vi "SetupControls.vi"(8 "Error IN":errorcluster, 11 "hCamera IN":u32) -> (0 "Error OUT":errorcluster, 3 "hCamera OUT":u32)   [LabVIEW 2013]
uses:
  Controls/Control References.ctl
  <vilib>/addons/PixeLINK/Low Level Functions/CAMERA_FEATURES.llb/TDPU-CameraFeatures-PixelAddressingMode.ctl
panel:
  in  "Camera Control References":T1
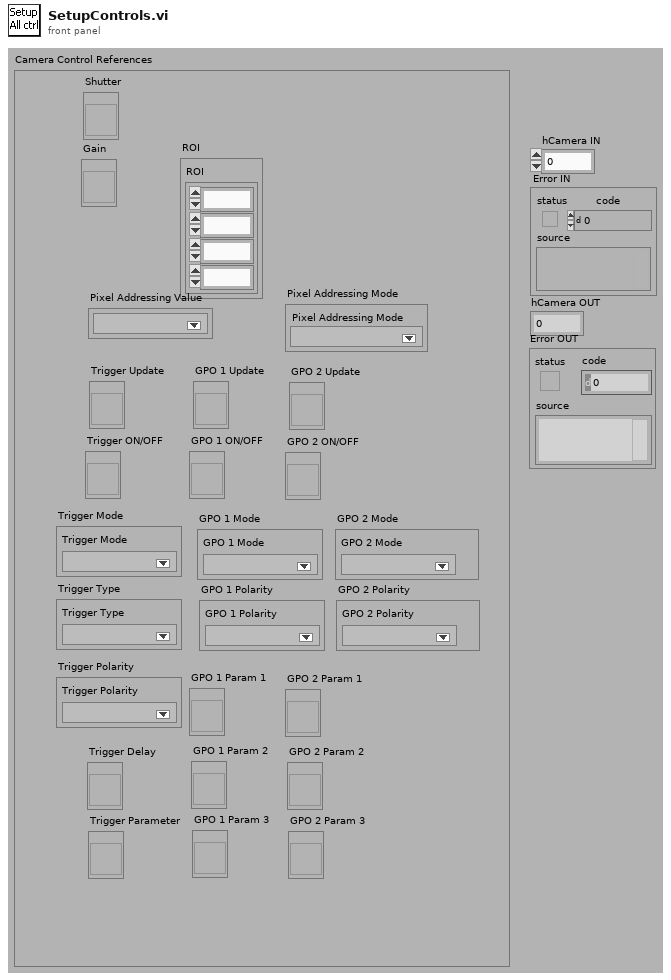
[diagram p1: front panel]
types:
  T1 = typedef "Control References.ctl" = cluster{"Shutter":refnum<vi>, "Gain":refnum<vi>, "ROI":refnum<vi>, "Pixel Addressing Value":refnum<vi>, "Trigger ON/OFF":refnum<vi>, "Trigger Mode":refnum<vi>, "Trigger Type":refnum<vi>, "Trigger Polarity":refnum<vi>, "Trigger Delay":refnum<vi>, "Trigger Parameter":refnum<vi>, "GPO 1 Mode":refnum<vi>, "GPO 1 Polarity":refnum<vi>, "GPO 1 Param 2":refnum<vi>, "GPO 1 Param 3":refnum<vi>, "GPO 1 Param 1":refnum<vi>, "GPO 1 ON/OFF":refnum<vi>, "GPO 2 Mode":refnum<vi>, "GPO 2 Polarity":refnum<vi>, "GPO 2 Param 2":refnum<vi>, "GPO 2 Param 3":refnum<vi>, "GPO 2 Param 1":refnum<vi>, "GPO 2 ON/OFF":refnum<vi>, "Trigger Update":refnum<vi>, "GPO 1 Update":refnum<vi>, "GPO 2 Update":refnum<vi>, "Pixel Addressing Mode":refnum<vi>}
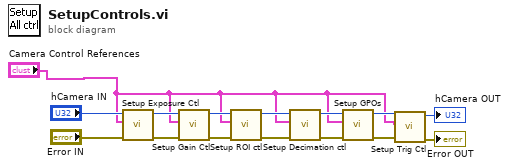
[diagram p0: block diagram]
diagram:
  n1 = call "Setup Exposure Ctl.vi"("Error IN"="Error IN", "PL-A741 Control References"="Camera Control References", "hCamera IN"="hCamera IN") -> ("Error OUT"=w4:errorcluster, "phCamera OUT"=w3:u32)  [unwired: 7 out]
  n2 = call "Setup Gain Ctl.vi"("Error IN"=w4, "PL-A741 Control References"="Camera Control References", "hCamera IN"=w3) -> ("Error OUT"=w7:errorcluster, "phCamera OUT"=w6:u32)  [unwired: 3 in, 4 out]
  n3 = call "Setup ROI ctl.vi"("Error IN"=w7, "PL-A741 Control References"="Camera Control References", "hCamera IN"=w6) -> ("Error OUT"=w9:errorcluster, "phCamera OUT"=w8:u32)  [unwired: 7 out]
  n4 = call "Setup Decimation ctl.vi"("Error IN"=w9, "PL-A741 Control References"="Camera Control References", "hCamera IN"=w8) -> ("Error OUT"=w11:errorcluster, "hCamera OUT"=w10:u32)  [unwired: 7 out]
  n5 = call "Setup GPOs.vi"("Error IN"=w11, "PL-A741 Control References"="Camera Control References", "hCamera IN"=w10) -> ("Error OUT"=w13:errorcluster, "hCamera OUT"=w12:u32)  [unwired: 7 out]
  n6 = call "Setup Trig Ctl.vi"("Error IN"=w13, "PL-A741 Control References"="Camera Control References", "hCamera IN"=w12) -> ("Error OUT"=→"Error OUT":errorcluster, "hCamera OUT"=→"hCamera OUT":u32)  [unwired: 7 out]
